vi "TS Acq Start.vi"(8 "error in":errorcluster, 11 "DeepU Test Stand in":refnum<class "DeepU Test Stand.lvclass">) -> (0 "error out":errorcluster, 3 "DeepU Test Stand out":refnum<class "DeepU Test Stand.lvclass">)   [LabVIEW 2019, in "Test Stands.lvlib" / "DeepU Test Stand.lvclass"]
uses:
  DeepU Test Stand.lvclass
  <vilib>/DAQmx/write.llb/DAQmx Write (Digital Bool 1Line 1Point).vi
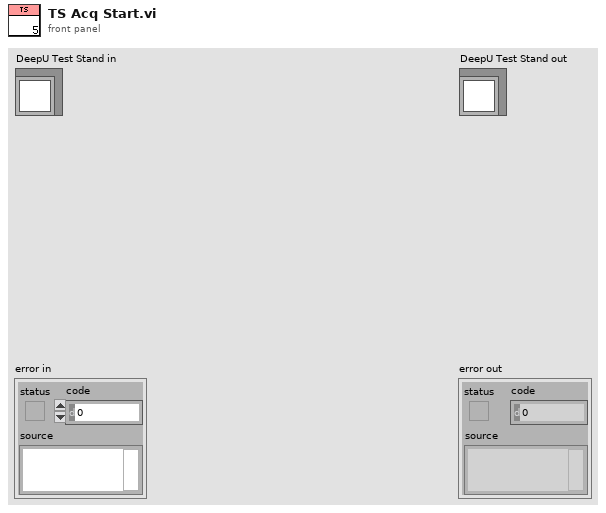
[diagram p1: front panel]
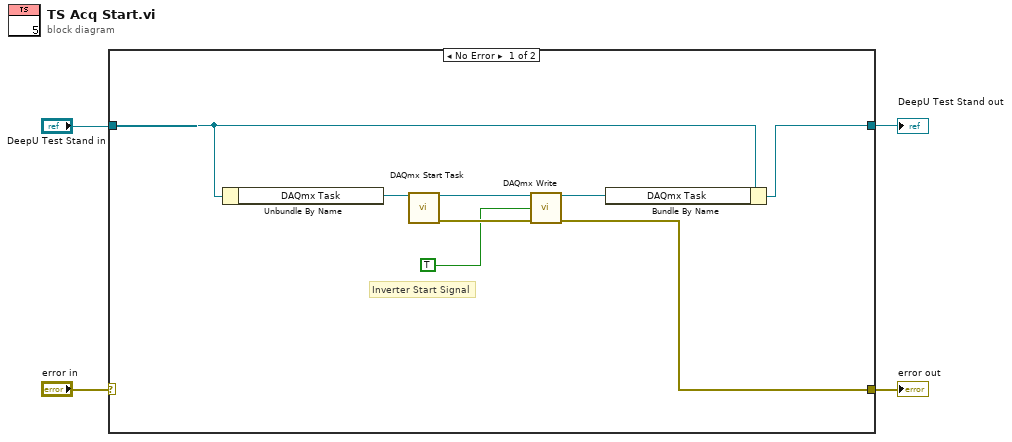
[diagram p0: block diagram]
diagram:
  n1 = case shown="No Error" "error in" {
    selector: "error in" -> [_ w14]
    tunnel: [w10 w14] -> w1
    tunnel: [w11 w13] -> w3
    tunnel: "DeepU Test Stand in" -> [w12 w13]
    frame No Error {
      # "Inverter Start Signal"
      n2 = Unbundle By Name(w12) -> ("DAQmx Task"=w9:refnum<k21>)
      n3 = call <vilib>:"DAQmx Start Task.vi"("task/channels in"=w9) -> ("task out"=w8:refnum<k21>, "error out"=w7:errorcluster)  [unwired: 13 in]
      n4 = call-poly <vilib>:"DAQmx Write.vi"("task/channels in"=w8, "data"=TRUE, "error in"=w7) -> ("task out"=w6:refnum<k21>, "error out"=w10:errorcluster)  [unwired: 10 in, 1 out]
      n5 = Bundle By Name(cluster=w12, "DAQmx Task"=w6) -> (w11:refnum<class "DeepU Test Stand.lvclass">)
    }
    frame Error {
    }
  }
  "error out" <- w1
  "DeepU Test Stand out" <- w3
